vi "MNIST_Optical_int_(SGD)_WB con__v2.2.vi"() -> ()   [LabVIEW 2021]
uses:
  <vilib>/Utility/file.llb/Write Delimited Spreadsheet (I64).vi
  <vilib>/Utility/file.llb/Write Delimited Spreadsheet (DBL).vi
  <vilib>/Utility/file.llb/Read Delimited Spreadsheet (I64).vi
panel:
  in  "WB convert?":bool
  in  "Save? (MiniBatch rows)":bool=TRUE
  in  "Add_in MNIST Rows":string="_MNIST_row_"
  in  "Save? (MiniBatch Num)":bool=TRUE
  in  "Add_in MNIST Num":string="_MNIST_Num_"
  out "Loss":ext
  in  "Save? (EL)":bool=TRUE
  in  "Add_in Erorrs":string="_Errors_"
  in  "Save? (AL)":bool=TRUE
  in  "Add_in Acc&Loss":string="_AL_"
  out "Loss":cluster{i32[], ext[]}(graph)={[1, 2], [45.514396123094795724, nan]}
  in  "Wait2 (ms)":u32=50
  out "Gaussian1 2":dbl[](graph)=[0.09670196140902938, 0.11442214309990176, 0.1351797003320732, 0.15945549418149738, 0.18779935795926087, 0.22083877294599188, 0.2592884397890202, 0.3039608080611435, 0.3557776262498078, 0.41578257333843466, 0.4851550310208827, 0.5652250523124651, 0.657489577737682, 0.7636299442341417, 0.8855307242605183, 1.0252999231821531, 1.1852905516835754, 1.3681235765830648, 1.5767122378728002, 1.8142877019668504, 2.08442600091682, 2.3910761846854314, 2.7385895884155467, 3.131750088996824, 3.57580519515535, 4.076497782861314, 4.640098253206141, 5.273436853240591, 5.983935861846952, 6.779641302867088, 7.669253806815572, 8.662158201039357, 9.768451366679242, 10.99896785985421, 12.365302754810589, 13.879831129103666, 15.555723576025287, 17.406957098330608, 19.448320710770176, 21.69541505796304, 24.164645339736463, 26.873206829207685, 29.83906227058617, 33.0809104548975, 36.61814529350236, 40.470804742262374, 44.65950897426188, 49.20538725679313, 54.12999305937387, 59.45520700425477, 65.20312736937558, 71.39594796601034, 78.05582333916168, 85.2047213776204, 92.86426357174314, 101.05555331939847, 109.79899285287111, 119.11408954021445, 129.01925250173178, 139.53158067379627, 150.66664364569763, 162.4382567879829, 174.85825237998242, 187.93624862685874, 201.6794186294016, 216.0922615296473, 231.1763781989189, 246.93025395874426, 263.3490509260849, 280.424412649283, 298.14428374720154, 316.49274727852463, 335.44988254878865, 354.99164600746684, 375.0897777948495, 395.7117363675348, 416.82066346163936, 438.37538144448484, 460.3304248592841, 482.63610768466145, 505.2386275137416, 528.0802075087822, 551.0992766102449, 574.2306880778159, 597.4059760197224, 620.5536491308751, 643.5995204154158, 666.4670712211182, 689.0778474680089, 711.3518855179752, 733.2081647125599, 754.5650832091166, 775.3409533774449, 795.4545126860733, 814.8254457153614, 833.3749126888666, 851.0260797197676, 867.7046458296478, 883.3393617159861, 897.8625352247819, 911.2105185274822, 923.3241721074656, 934.149300830448, 943.6370576040389, 951.7443104220167, 958.4339689354637, 963.6752670915627, 967.4439988266017, 969.7227042867535, 970.5008045720157, 969.7746835482575, 967.5477158420546, 963.8302407150543, 958.6394821008861, 951.9994156699714, 943.9405843578882, 934.4998643433248, 923.7201839845574, 911.6501987117265, 898.3439253194533, 883.8603395047159, 868.2629408433546, 851.6192896909191, 834.0005207265273, 815.4808380296865, 796.1369966882987, 776.0477759809958, 755.2934491591791, 733.9552547752518, 712.1148743660126, 689.8539211073784, 667.253443812555, 644.3934503552997, 621.3524542682865, 598.2070478996438, 575.0315051146013, 551.8974161102901, 528.873356476583, 506.0245921909981, 483.4128217875633, 461.0959564943735, 439.1279386983413, 417.5585986738939, 396.43354911021174, 375.7941165936193, 355.6773088519376, 336.115816249367, 317.1380457365506, 298.7681852129464, 281.0262960489612, 263.9284313442493, 247.48677736631487, 231.709815519667, 216.60250213925784, 202.16646338132895, 188.4002024981488, 175.2993168281445, 162.85672190694973, 151.06288020502143, 139.9060321206019, 129.37242699969255, 119.44655211405521, 110.11135770074489, 101.3484763490417, 93.13843520969536, 85.46085969410542, 78.29466752455427, 71.61825218825167, 65.40965503532775, 59.646725441864234, 54.30726863171807, 49.36918091364827, 44.810572241806135, 40.60987614694352, 36.745947211971774, 33.19814637826082, 29.94641446804717, 26.971334393482046, 24.254182594381085, 21.776970304983546, 19.522475295517197, 17.474264767749766, 15.616710105755313, 13.934994194693601, 12.41511202241696, 11.043865272147123, 9.80885160030031, 8.69844927277758, 7.701797806667482, 6.8087752332916445, 6.009972563782131, 5.296666000789356, 4.660787400295918, 4.094893446609467, 3.5921339621107853, 3.1462197318544955, 2.751390182199411, 2.4023812127511532, 2.0943934424259196, 1.8230610937190317]
  out "Gaussian1":dbl[](graph)=[0.5699152503773883, 0.6314492251008037, 0.6989600685377171, 0.7729511904764719, 0.853960042130039, 0.9425595629244234, 1.0393596017692057, 1.1450083015934553, 1.2601934350188855, 1.3856436781332593, 1.5221298084293, 1.6704658120969746, 1.831509885009732, 2.0061653109390867, 2.1953811997776564, 2.400153067860802, 2.6215232418633736, 2.8605810672237024, 3.1184629016252225, 3.3963518737600005, 3.695477387421891, 4.017114350943006, 4.362582112109385, 4.733243078982677, 5.130501007526851, 5.555798937604037, 6.0106167597722555, 6.496468396399691, 7.014898581913567, 7.567479228533548, 8.155805365605005, 8.781490642649525, 9.446162388490219, 10.15145622128628, 10.899010207021403, 11.690458566928344, 12.527424937487345, 13.41151518999903, 14.344309820286899, 15.327355922814016, 16.362158767381846, 17.450173000593374, 18.5927934983811, 19.791345900093123, 21.047076858867005, 22.361144047264876, 23.73460596135841, 25.168411570599666, 26.66338986485152, 28.220239353838334, 29.839517577968138, 31.521630692929637, 33.266823193633265, 35.0751678459036, 36.94655589679441, 38.88068763644488, 40.877063385986645, 42.93497498710372, 45.05349786940917, 47.23148377179553, 49.46755419331591, 51.760094647931396, 54.10724979559787, 56.506919519648946, 58.95675601724929, 61.45416196584334, 63.996289824009004, 66.58004231995741, 69.20207417511158, 71.85879510377347, 74.54637412288272, 77.26074519831532, 79.99761424611384, 82.75246749853183, 85.52058123587125, 88.29703287585642, 91.07671340279033, 93.85434110905102, 96.62447661168733, 99.38153909704506, 102.11982373658174, 104.83352020739565, 107.51673224159532, 110.16349811954991, 112.7678120133866, 115.32364607891411, 117.82497318654511, 120.26579017483816, 122.64014150406159, 124.94214318176782, 127.16600682782045, 129.30606374269755, 131.35678884025123, 133.3128243044793, 135.1690028292909, 136.92037030074718, 138.5622077828464, 140.09005267059928, 141.49971887790022, 142.78731593252587, 143.94926685645228, 144.98232471654234, 145.8835877384628, 146.65051288539, 147.28092781258692, 147.77304111920574, 148.12545082960688, 148.33715104799708, 148.40753674217896, 148.3364066245716, 148.12396411130277, 147.7708163529763, 147.27797134357863, 146.6468331267909, 145.87919513161353, 144.9772316815739, 143.94348773377754, 142.78086691557044, 141.49261793751415, 140.08231947164353, 138.5538635934956, 136.911437895094, 135.1595063838758, 133.30278928940297, 131.34624190555502, 129.29503260072028, 127.15452013225598, 124.93023040416011, 122.6278328084785, 120.2531162914655, 117.81196528493653, 115.31033564162118, 112.75423071067677, 110.14967768589845, 107.50270435461167, 104.81931636981285, 102.10547516190402, 99.36707659940957, 96.60993050045434, 93.83974108859331, 91.06208847790437, 88.28241126317056, 85.50599028157492, 82.73793360269933, 79.98316279384422, 77.24640049785856, 74.53215935087066, 71.8447322576235, 69.1881840326221, 66.56634440606591, 63.98280238463786, 61.4409019487149, 58.943739059510534, 56.494159942108, 54.09476060333887, 51.74788753704222, 49.45563956343463, 47.21987074415553, 45.04219431004106, 42.92398753483382, 40.866397484856755, 38.87034757216636, 36.936544836841676, 35.065487882847584, 33.25747539131333, 31.51261513506436, 29.830833418809526, 28.211884870481356, 26.655362510820165, 25.16070803034281, 23.727222205302944, 22.35407538708896, 21.040318002674137, 19.78489100718638, 18.586636233356952, 17.444306586495248, 16.3565760376754, 15.322049371967854, 14.339271652764877, 13.40673736749281, 12.522899224239719, 11.686176573019994, 10.894963429515084, 10.14763608314326, 9.442560275193749, 8.778097936489429, 8.152613477595633, 7.564479627954442, 7.012082823478275, 6.493828145073044, 6.008143813270019, 5.553485246621279, 5.128338693752555, 4.731224450967974, 4.360699679065516, 4.015360834552515, 3.6938457317528375, 3.394835253378139, 3.117054728003027, 2.8592749935482025, 2.620313166346684, 2.3990331356583474, 2.194345803619269, 2.005209090577634, 1.8306277255905967, 1.6696528415498544, 1.521381393981185, 1.3849554220385487, 1.259561169599107, 1.1444280836752243, 1.0388277066049971, 0.9420724776763157, 0.8535144589920913, 0.7725439995066742, 0.6985883502657112, 0.6311102429727983, 0.569606443094855, 0.5136062878118027, 0.46267021822177495, 0.4163883143369015, 0.3743788405519984, 0.33628680844400993, 0.3017825629676108, 0.270560397355318, 0.24233720131135278, 0.21685114640935305, 0.1938604119662967, 0.17314195406955885, 0.15449031988137882, 0.13771650883509554, 0.12264688187001148, 0.10912211942590293, 0.09699622853300671, 0.08613559898751195, 0.07641810829465917, 0.06773227478986307, 0.05997645811098017, 0.053058105990058196, 0.04689304615861079, 0.04140482201462393, 0.03652407058005483, 0.03218794118245605, 0.028339553221509016, 0.02492749132866501, 0.021905336193819215, 0.01923122931509139, 0.016867469924549863, 0.014780142352357088, 0.012938772112715328, 0.011316009025602454]
  in  "SGD?":bool
  in  "Save? (SP)":bool=TRUE
  in  "Add_in Spectrum":string="_spectrum_"
  out "Accuracy(current)":dbl=0.3076923076923077
  out "Errors(current)":i32=36
  out "weight No.":i32=7
  out "epoch":i32=2
  out "Output (Converted)":dbl[](graph)=[39.62523093192144, 0.0, 23.097154266476934, 78.25935170802192, 80.61297751490206, 88.079328272374, 139.1328670628771, 91.58552612543261, 147.85235008560898, 50.15605743167636]
  out "from Start Acq":u32=20002
  out "Waveform Graph 0":i32[](graph)=[148, 148, 147, 146, 147, 147, 149, 149, 148, 148, 146, 147, 146, 149, 148, 148, 148, 149, 148, 147, 148, 147, 148, 146, 150, 149, 148, 147, 148, 147, 148, 148, 147, 149, 147, 145, 149, 148, 148, 146, 148, 148, 146, 148, 150, 150, 147, 148, 150, 147, 146, 148, 148, 147, 146, 151, 151, 153, 149, 149, 148, 150, 149, 151, 152, 151, 149, 149, 150, 150, 150, 150, 150, 154, 150, 152, 153, 152, 152, 152, 155, 155, 153, 154, 156, 155, 156, 159, 159, 161, 163, 161, 161, 163, 161, 165, 168, 168, 167, 169, 172, 178, 175, 176, 179, 178, 184, 186, 186, 188, 190, 194, 200, 200, 200, 200, 206, 205, 207, 212, 220, 222, 219, 221, 227, 231, 234, 233, 237, 244, 247, 246, 253, 257, 262, 259, 266, 270, 273, 279, 279, 281, 280, 284, 292, 291, 301, 297, 298, 301, 307, 303, 300, 306, 303, 309, 307, 305, 303, 307, 303, 307, 300, 301, 295, 288, 291, 289, 286, 280, 279, 280, 271, 270, 264, 268, 264, 260, 262, 251, 250, 251, 248, 241, 236, 240, 233, 230, 230, 232, 225, 224, 225, 220, 223, 219, 216, 221, 213, 212, 205, 210, 206, 202, 203, 201, 203, 198, 197, 202, 194, 195, 193, 196, 187, 191, 188, 187, 184, 183, 184, 181, 181, 178, 178, 179, 178, 173, 176, 175, 177, 174, 171, 174, 170, 172, 171, 170, 168, 166, 169, 169, 168, 163, 167, 165, 162, 162, 164, 163, 163, 162, 161, 163, 159, 161, 163, 162, 159, 157, 156, 157, 156, 158, 158, 155, 155, 153, 155, 156, 154, 155, 155, 151, 151, 153, 151, 152, 151, 150, 150, 151, 150, 151, 151, 151, 151, 150, 148, 151, 148, 150, 149, 149, 149, 149, 148, 149, 148, 148, 150, 150, 150, 149, 149, 150, 150, 149, 148, 152, 150, 150, 149, 148, 150, 149, 150, 147, 150, 151, 150, 150, 149, 149, 147, 149, 147, 149, 149, 149, 148, 151, 150, 148, 149, 150, 151, 149, 149, 150, 152, 150, 150, 150, 148, 148, 148, 149, 149, 147, 147, 148, 150, 150, 148, 149, 149, 149, 148, 149, 147, 149, 152, 149, 148, 150, 149, 149, 150, 150, 150, 148, 151, 150, 150, 148, 150, 149, 150, 147, 149, 152, 150, 148, 149, 148, 150, 149, 149, 149, 149, 150, 149, 149, 151, 148, 150, 150, 152, 149, 151, 151, 149, 146, 150, 148, 148, 149, 150, 148, 149, 150, 148, 149, 148, 150, 148, 150, 150, 149, 150, 150, 147, 152, 148, 150, 150, 149, 151, 149, 150, 148, 149, 149, 149, 149, 148, 147, 150, 149, 149, 151, 151, 151, 148, 150, 148, 150, 151, 149, 149, 147, 151, 150, 147, 149, 149, 150, 150, 149, 149, 151, 149, 149, 149, 150, 148, 152, 149, 150, 150, 151, 149, 149, 149, 148, 149, 149, 149, 149, 148, 149, 148, 149, 150, 150, 148, 149, 150, 149, 149, 148, 151, 150, 149, 151, 148, 148, 149, 147, 150, 151, 148, 151, 150, 150, 149, 148, 149, 150, 150, 149, 149, 151, 148, 148, 151, 151, 148, 148, 149, 150, 151, 149, 151, 152, 151, 151, 150, 151, 151, 151, 149, 148, 148, 150, 152, 152, 148, 152, 151, 151, 150, 150, 151, 151, 151, 151, 153, 152, 151, 153, 153, 152, 153, 155, 153, 154, 155, 151, 153, 156, 154, 154, 154, 156, 155, 156, 157, 158, 155, 157, 158, 160, 159, 159, 160, 161, 162, 163, 165, 166, 164, 170, 169, 169, 171, 172, 176, 174, 174, 178, 181, 183, 185, 187, 186, 193, 196, 194, 199, 199, 202, 203, 210, 211, 219, 219, 221, 226, 233, 237, 242, 246, 252, 257, 260, 269, 274, 277, 281, 287, 292, 303, 309, 313, 327, 328, 340, 346, 359, 367, 371, 377, 389, 402, 406, 418, 437, 436, 447, 453, 463, 480, 488, 500, 519, 530, 523, 550, 570, 597, 601, 605, 622, 639, 646, 660, 684, 691, 711, 736, 760, 767, 795, 792, 827, 838, 864, 877, 898, 912, 934, 946, 980, 991, 1021, 1041, 1053, 1067, 1064, 1089, 1100, 1120, 1125, 1134, 1153, 1155, 1150, 1134, 1151, 1151, 1142, 1126, 1109, 1108, 1100, 1069, 1045, 1015, 987, 971, 934, 904, 875, 844, 816, 793, 760, 731, 704, 680, 651, 619, 587, 575, 549, 516, 510, 488, 473, 456, 436, 414, 403, 393, 381, 357, 348, 339, 329, 324, 311, 299, 292, 286, 276, 271, 267, 257, 253, 246, 241, 231, 233, 227, 224, 216, 214, 209, 209, 202, 201, 200, 197, 195, 191, 186, 187, 184, 184, 179, 180, 178, 173, 176, 176, 169, 174, 169, 167, 170, 167, 171, 167, 167, 166, 164, 164, 161, 162, 161, 161, 158, 161, 157, 160, 157, 160, 157, 155, 157, 156, 155, 156, 155, 155, 155, 153, 154, 154, 153, 154, 155, 154, 154, 154, 152, 152, 153, 150, 152, 154, 153, 153, 150, 152, 152, 150, 150, 153, 150, 149, 149, 151, 151, 151, 151, 150, 151, 150, 150, 151, 152, 150, 148, 150, 152, 151, 150, 149, 149, 150, 149, 151, 148, 150, 150, 149, 149, 150, 148, 151, 151, 148, 149, 150, 150, 149, 149, 149, 149, 151, 147, 149, 149, 149, 146, 151, 151, 150, 148, 147, 151, 149, 149, 147, 151, 147, 148, 150, 147, 148, 148, 149, 150, 147, 148, 148, 150, 148, 150, 148, 149, 148, 150, 148, 147, 147, 146, 150, 149, 149, 150, 147, 150, 149, 148, 150, 149, 149, 148, 148, 149, 148, 147, 149, 149, 147, 149, 148, 147, 146, 149, 148, 149, 147, 147, 147, 149, 148, 147, 149, 149, 150, 147, 147, 149, 151, 150, 148, 148, 148, 146, 147, 149, 148, 146, 149, 148, 147, 149, 147, 148, 149, 149, 147, 147, 148, 149, 149, 146, 149, 147, 150, 147, 148, 149, 149, 148, 149, 148, 149, 148, 148, 150, 148, 149, 148, 147, 148, 147, 147, 149, 148, 149, 148, 147, 148, 147, 148, 148, 147, 149, 148, 147, 148, 150, 148, 147, 147, 150, 147, 147, 147, 148, 148, 149, 149, 147, 146, 147, 149, 150, 147, 146, 149, 149, 148, 146, 146, 149, 147, 148]
  in  "Ind1":i32=50
  in  "Leng1":i32=250
  in  "Ind2":i32=575
  in  "Leng2":i32=200
  in  "Compen_Factor":dbl=3.0
  out "In * W (i) +B (i)":dbl[][](graph)
  in  "Wait1 (ms)":u32=50
  out "Weights(i)":dbl[][](graph)=[[25.0, 75.0, 53.0, -76.0, -17.0, -21.0, -83.0, 41.0, -26.0, -83.0, -71.0, -83.0, 76.0, -65.0, 57.0, 83.0, -8.0, 41.0, -28.0, 67.0, 47.0, 31.0, -41.0, 72.0, -83.0, 81.0, -16.0, -24.0], [5.0, -71.0, 45.0, 74.0, 50.0, -18.0, -76.0, 28.0, -37.0, -41.0, -28.0, 2.0, -20.0, -69.0, 53.0, 83.0, 10.0, -70.0, 83.0, -53.0, -49.0, 56.0, 53.0, -3.0, -83.0, -57.0, -76.0, 56.0], [44.0, -79.0, 83.0, 51.0, 30.0, 46.0, 12.0, 41.0, 3.0, -20.0, -50.0, 83.0, -50.0, 83.0, -36.0, -65.0, -76.0, -52.0, 25.0, -17.0, 21.0, 23.0, -29.0, 15.0, 80.0, 70.0, 19.0, -83.0], [-65.0, -83.0, -83.0, 38.0, -7.0, 41.0, 44.0, 50.0, 80.0, 23.0, 34.0, -5.0, 83.0, -12.0, 0.0, -14.0, -2.0, -25.0, -83.0, 40.0, -62.0, -83.0, 56.0, -83.0, 83.0, -4.0, 48.0, 25.0], [-83.0, -83.0, 65.0, -41.0, -71.0, -81.0, -8.0, -45.0, 41.0, -76.0, -32.0, -56.0, 41.0, -78.0, -83.0, -83.0, 23.0, -74.0, 17.0, -15.0, -72.0, 41.0, -83.0, 41.0, 44.0, 83.0, -57.0, -83.0], [-83.0, -28.0, 8.0, 81.0, 71.0, 78.0, -3.0, -79.0, -10.0, -83.0, -21.0, 10.0, 21.0, -86.0, -8.0, -56.0, -3.0, -90.0, -25.0, -52.0, -2.0, 19.0, -43.0, -59.0, 49.0, 83.0, 37.0, -28.0], [5.0, 52.0, -83.0, -12.0, -34.0, 32.0, -42.0, -53.0, -50.0, -87.0, -52.0, -18.0, -89.0, 76.0, -26.0, 10.0, 23.0, 5.0, -83.0, -33.0, 36.0, -60.0, 1.0, -32.0, -83.0, 83.0, -58.0, -12.0], [17.0, -41.0, -59.0, 38.0, -8.0, 39.0, 71.0, -15.0, 76.0, 18.0, 87.0, -78.0, -6.0, 75.0, 49.0, -43.0, 25.0, 39.0, 58.0, -42.0, -76.0, -83.0, -9.0, 83.0, 55.0, -21.0, -83.0, 23.0], [-83.0, -83.0, 29.0, 81.0, 36.0, 94.0, 20.0, 106.0, 38.0, 1.0, 99.0, 90.0, -25.0, 10.0, 107.0, 70.0, 91.0, 101.0, -3.0, 103.0, -14.0, -34.0, -83.0, -58.0, 1.0, -83.0, -5.0, 11.0], [65.0, 85.0, 25.0, 83.0, 32.0, 24.0, -65.0, 43.0, -29.0, 93.0, 108.0, -15.0, 26.0, 103.0, 50.0, 115.0, 125.0, 75.0, 113.0, -17.0, 6.0, -37.0, -28.0, -83.0, 36.0, -7.0, 62.0, -8.0], [56.0, -36.0, 80.0, -32.0, 64.0, 35.0, 90.0, 25.0, 52.0, 87.0, 106.0, 72.0, 101.0, -59.0, 47.0, 115.0, 110.0, 71.0, 106.0, 113.0, 81.0, 98.0, 86.0, -63.0, 83.0, 83.0, 36.0, 33.0], [24.0, 6.0, 9.0, -41.0, 50.0, -18.0, 56.0, 65.0, 87.0, -42.0, 103.0, 19.0, 28.0, -79.0, -17.0, 83.0, 48.0, 112.0, 110.0, 99.0, 66.0, 95.0, 5.0, -18.0, -77.0, -41.0, -71.0, 83.0], [9.0, -36.0, 26.0, 83.0, 41.0, 5.0, 39.0, -17.0, 101.0, -13.0, 45.0, 50.0, -69.0, -74.0, -10.0, -40.0, -12.0, -32.0, 65.0, -11.0, 41.0, -37.0, 23.0, 40.0, 0.0, 23.0, 62.0, -80.0], [40.0, -39.0, 83.0, 74.0, -61.0, 6.0, -14.0, -1.0, -9.0, 53.0, -14.0, -158.0, -125.0, -96.0, 32.0, 9.0, -63.0, 60.0, -32.0, -23.0, 74.0, 26.0, 74.0, 83.0, 83.0, -42.0, -56.0, 83.0], [-83.0, -3.0, 67.0, 59.0, 26.0, 82.0, 2.0, 84.0, 15.0, -87.0, -90.0, -135.0, -113.0, -92.0, -58.0, -24.0, 77.0, 109.0, -13.0, 94.0, -12.0, 38.0, 32.0, -3.0, 40.0, 35.0, -35.0, 17.0], [81.0, 37.0, 38.0, 30.0, -37.0, 34.0, 3.0, -54.0, 59.0, -98.0, -31.0, -60.0, -127.0, -45.0, -70.0, 20.0, 76.0, 61.0, 40.0, -8.0, -32.0, 35.0, -76.0, 46.0, 86.0, -50.0, -17.0, 83.0], [28.0, -53.0, 19.0, 18.0, -78.0, 3.0, 65.0, -59.0, 85.0, 86.0, -32.0, -40.0, 0.0, 41.0, -46.0, 68.0, 21.0, 97.0, 99.0, -65.0, -65.0, 4.0, -6.0, -83.0, -83.0, 75.0, 0.0, 61.0], [65.0, -83.0, 78.0, -44.0, -41.0, -83.0, -33.0, -63.0, 7.0, 25.0, -76.0, -22.0, -16.0, -2.0, 124.0, 15.0, 50.0, -68.0, -14.0, 68.0, -87.0, -55.0, -81.0, -26.0, 2.0, -65.0, 19.0, -14.0], [15.0, -41.0, -15.0, -68.0, -55.0, 39.0, 74.0, -52.0, 79.0, -37.0, -71.0, -8.0, -15.0, 95.0, 88.0, 70.0, 12.0, 41.0, -52.0, 43.0, -86.0, -87.0, -85.0, -64.0, 41.0, -80.0, 23.0, -79.0], [69.0, 25.0, -65.0, 83.0, 33.0, -32.0, -83.0, -36.0, -80.0, -36.0, 18.0, 37.0, -15.0, 36.0, 38.0, 110.0, -45.0, -80.0, -57.0, 31.0, -19.0, -22.0, -56.0, 83.0, -83.0, 3.0, -28.0, -83.0], [-35.0, 83.0, 74.0, 38.0, -26.0, 83.0, 48.0, 44.0, -83.0, 65.0, 46.0, -24.0, 12.0, 23.0, -58.0, 25.0, -29.0, -49.0, 41.0, 42.0, 38.0, -57.0, 11.0, 17.0, -76.0, -15.0, -48.0, 72.0], [83.0, -83.0, -67.0, -57.0, 83.0, 83.0, -79.0, -14.0, 72.0, -78.0, -71.0, -74.0, -26.0, 98.0, 103.0, -28.0, -20.0, 17.0, -85.0, -17.0, -85.0, -54.0, -85.0, -17.0, -57.0, 6.0, -80.0, -76.0], [-83.0, 67.0, 64.0, -56.0, 76.0, 71.0, 46.0, -69.0, -37.0, 68.0, 14.0, 19.0, -32.0, -35.0, -37.0, 55.0, 11.0, -46.0, 19.0, -28.0, 30.0, -8.0, 60.0, 9.0, 41.0, 36.0, -31.0, -83.0], [42.0, 57.0, -50.0, 83.0, -71.0, -72.0, 83.0, 0.0, 87.0, -57.0, 48.0, 91.0, -76.0, -40.0, 5.0, 62.0, -50.0, -79.0, -25.0, -41.0, 32.0, 1.0, 83.0, 6.0, -83.0, -52.0, -72.0, 7.0], [41.0, 53.0, -76.0, -74.0, 62.0, -44.0, -1.0, 52.0, 20.0, 85.0, 92.0, 41.0, 54.0, 9.0, 114.0, 82.0, -81.0, 46.0, -49.0, -79.0, -74.0, 43.0, -28.0, -83.0, 26.0, -30.0, 83.0, 83.0], [-57.0, -83.0, 23.0, 52.0, -25.0, 49.0, -28.0, 22.0, -34.0, 42.0, 32.0, -11.0, 82.0, 99.0, 99.0, -25.0, 58.0, 52.0, -65.0, 83.0, 53.0, 32.0, 56.0, -43.0, 61.0, 25.0, -83.0, -32.0], [-77.0, 83.0, 80.0, 37.0, 33.0, -83.0, 3.0, 24.0, 90.0, -17.0, -45.0, -78.0, 97.0, 80.0, 36.0, 73.0, 53.0, 68.0, 83.0, -41.0, 83.0, -66.0, -83.0, 14.0, -79.0, 59.0, -83.0, 83.0], [-35.0, -83.0, 48.0, 78.0, 47.0, 13.0, -79.0, 30.0, -64.0, -5.0, 36.0, -39.0, 50.0, -26.0, -83.0, -8.0, -51.0, -25.0, 77.0, -56.0, 21.0, -83.0, -11.0, -41.0, -41.0, 57.0, 81.0, -44.0], [-71.0, 0.0, 0.0, 0.0, 0.0, 0.0, 0.0, 0.0, 0.0, 0.0, 0.0, 0.0, 0.0, 0.0, 0.0, 0.0, 0.0, 0.0, 0.0, 0.0, 0.0, 0.0, 0.0, 0.0, 0.0, 0.0, 0.0, 0.0]]
  in  "WB Import?":bool=TRUE
  out "Output (Measured)":dbl[](graph)=[792.5046186384288, -931.6896199556032, 461.9430853295387, 1565.1870341604385, 1612.2595502980412, 1761.58656544748, 2782.6573412575417, 1831.710522508652, 2957.0470017121793, 1003.1211486335272]
  in  "Epochs":i64=200
  out "Accu":cluster{i32[], dbl[]}(graph)={[1, 2], [0.29, 0.14]}
  in  "Training rate":dbl=2.0 format="%#_13g"
  in  "Con.F":i32=20
  out "min value":i32=-255
  out "max value":i32=176
  in  "Add_in WB":string="_epoch__"
  out "W&B(int)":i32[][](array[numeric])
  out "Output (simulated)":dbl[](graph)=[-161692.0, -526023.0, -407243.0, 774561.0, -189118.0, -52721.0, -448721.0, 622480.0, 408514.0, -270311.0]
  out "Output (SoftMax)":ext[](graph)=[9.942335489197921718e-48, 6.1442556256622408318e-65, 6.5983587063865749592e-55, 5.9713685974966820238e-31, 6.2840637228245183395e-30, 1.0985896780412405855e-26, 0.000163344942582687903655, 3.6606473610987689061e-25, 0.99983665505741731205, 3.7236448483001870884e-43]
  out "No. Tested":i32=53
  out "Accuracy (prev)":dbl=0.14
  out "Errors":i32=86
  out "Error list":i32[][](array[numeric])=[[0, 2, 3, 5, 6, 7, 8, 9, 10, 11, 12, 13, 14, 15, 16, 17, 18, 20, 22, 23, 24, 25, 26, 27, 28, 29, 30, 31, 32, 33, 34, 35, 36, 38, 39, 40, 41, 42, 43, 44, 45, 46, 47, 48, 49, 50, 52, 53, 54, 55, 57, 58, 59, 60, 61, 62, 64, 65, 66, 67, 70, 71, 72, 73, 74, 76, 77, 78, 79, 80, 82, 83, 84, 85, 86, 87, 89, 90, 91, 92, 93, 94, 96, 97, 98, 99], [5, 4, 1, 2, 1, 3, 1, 4, 3, 5, 3, 6, 1, 7, 2, 8, 6, 4, 9, 1, 1, 2, 4, 3, 2, 7, 3, 8, 6, 9, 0, 5, 6, 7, 6, 1, 8, 7, 9, 3, 9, 8, 5, 9, 3, 3, 7, 4, 9, 8, 9, 4, 1, 4, 4, 6, 4, 5, 6, 1, 1, 7, 1, 6, 3, 2, 1, 1, 7, 9, 2, 6, 7, 8, 3, 9, 4, 6, 7, 4, 6, 8, 7, 8, 3, 1], [0, 0, 9, 0, 9, 0, 9, 9, 0, 1, 0, 0, 9, 0, 0, 1, 1, 9, 1, 9, 0, 8, 9, 0, 0, 9, 0, 9, 0, 0, 1, 0, 1, 0, 0, 9, 1, 9, 0, 0, 0, 9, 1, 0, 0, 0, 0, 9, 0, 9, 0, 9, 9, 9, 9, 1, 0, 1, 1, 9, 0, 0, 9, 1, 0, 1, 9, 9, 0, 0, 0, 0, 0, 1, 0, 0, 0, 0, 0, 0, 9, 9, 0, 1, 0, 9]]
  out "Match?":bool
  in  "Train No.":i32=10
  out "OUTPUT":i16=8
  out "MNIST_Input":i32[][](graph)=[[0, 0, 0, 0, 0, 0, 0, 0, 0, 0, 0, 0, 0, 0, 0, 0, 0, 0, 0, 0, 0, 0, 0, 0, 0, 0, 0, 0], [0, 0, 0, 0, 0, 0, 0, 0, 0, 0, 0, 0, 0, 0, 0, 0, 0, 0, 0, 0, 0, 0, 0, 0, 0, 0, 0, 0], [0, 0, 0, 0, 0, 0, 0, 0, 0, 0, 0, 0, 0, 0, 0, 0, 0, 0, 0, 0, 0, 0, 0, 0, 0, 0, 0, 0], [0, 0, 0, 0, 0, 0, 0, 0, 0, 0, 0, 0, 0, 0, 0, 0, 0, 0, 0, 0, 0, 0, 0, 0, 0, 0, 0, 0], [0, 0, 0, 0, 0, 0, 0, 0, 0, 0, 0, 0, 0, 0, 0, 0, 0, 0, 0, 0, 0, 0, 0, 0, 0, 0, 0, 0], [0, 0, 0, 0, 0, 0, 0, 0, 0, 0, 0, 0, 0, 0, 0, 0, 0, 0, 0, 0, 0, 0, 0, 0, 0, 0, 0, 0], [0, 0, 0, 0, 0, 0, 0, 0, 0, 0, 0, 0, 0, 0, 0, 0, 0, 0, 0, 0, 0, 0, 0, 0, 0, 0, 0, 0], [0, 0, 0, 0, 0, 0, 0, 1, 109, 109, 109, 109, 110, 109, 129, 253, 110, 109, 31, 0, 0, 0, 0, 0, 0, 0, 0, 0], [0, 0, 0, 0, 0, 21, 94, 217, 252, 252, 252, 252, 253, 252, 252, 252, 253, 252, 227, 134, 42, 0, 0, 0, 0, 0, 0, 0], [0, 0, 0, 0, 0, 176, 252, 252, 252, 252, 252, 252, 253, 252, 252, 252, 253, 252, 252, 252, 222, 139, 11, 0, 0, 0, 0, 0], [0, 0, 0, 0, 0, 217, 252, 252, 252, 128, 108, 108, 108, 108, 108, 108, 108, 232, 252, 252, 253, 252, 71, 0, 0, 0, 0, 0], [0, 0, 0, 0, 0, 42, 159, 252, 252, 210, 31, 0, 0, 0, 0, 0, 0, 0, 37, 252, 253, 252, 71, 0, 0, 0, 0, 0], [0, 0, 0, 0, 0, 0, 5, 119, 210, 252, 124, 31, 0, 0, 0, 0, 0, 0, 37, 252, 253, 231, 51, 0, 0, 0, 0, 0], [0, 0, 0, 0, 0, 0, 0, 0, 31, 195, 195, 31, 0, 0, 0, 0, 0, 0, 140, 252, 253, 158, 0, 0, 0, 0, 0, 0], [0, 0, 0, 0, 0, 0, 0, 0, 0, 0, 0, 0, 0, 0, 0, 0, 0, 42, 221, 252, 191, 15, 0, 0, 0, 0, 0, 0], [0, 0, 0, 0, 0, 0, 0, 0, 0, 0, 0, 0, 0, 0, 0, 0, 0, 218, 253, 253, 84, 0, 0, 0, 0, 0, 0, 0], [0, 0, 0, 0, 0, 0, 0, 0, 0, 0, 0, 0, 0, 0, 0, 0, 94, 247, 252, 210, 0, 0, 0, 0, 0, 0, 0, 0], [0, 0, 0, 0, 0, 0, 0, 0, 0, 0, 0, 0, 0, 0, 0, 21, 212, 252, 226, 31, 0, 0, 0, 0, 0, 0, 0, 0], [0, 0, 0, 0, 0, 0, 0, 0, 0, 0, 0, 0, 0, 0, 0, 144, 253, 252, 132, 0, 0, 0, 0, 0, 0, 0, 0, 0], [0, 0, 0, 0, 0, 0, 0, 0, 0, 0, 0, 0, 0, 0, 99, 253, 255, 222, 41, 0, 0, 0, 0, 0, 0, 0, 0, 0], [0, 0, 0, 0, 0, 0, 0, 0, 0, 0, 0, 0, 0, 21, 201, 252, 253, 55, 0, 0, 0, 0, 0, 0, 0, 0, 0, 0], [0, 0, 0, 0, 0, 0, 0, 0, 0, 0, 0, 0, 0, 94, 252, 252, 175, 10, 0, 0, 0, 0, 0, 0, 0, 0, 0, 0], [0, 0, 0, 0, 0, 0, 0, 0, 0, 0, 0, 0, 0, 217, 252, 252, 62, 0, 0, 0, 0, 0, 0, 0, 0, 0, 0, 0], [0, 0, 0, 0, 0, 0, 0, 0, 0, 0, 0, 0, 171, 253, 253, 170, 110, 78, 0, 0, 0, 0, 0, 0, 0, 0, 0, 0], [0, 0, 0, 0, 0, 0, 0, 0, 0, 0, 0, 0, 253, 252, 252, 252, 253, 55, 0, 0, 0, 0, 0, 0, 0, 0, 0, 0], [0, 0, 0, 0, 0, 0, 0, 0, 0, 0, 0, 0, 253, 252, 252, 252, 154, 10, 0, 0, 0, 0, 0, 0, 0, 0, 0, 0], [0, 0, 0, 0, 0, 0, 0, 0, 0, 0, 0, 0, 253, 252, 252, 168, 0, 0, 0, 0, 0, 0, 0, 0, 0, 0, 0, 0], [0, 0, 0, 0, 0, 0, 0, 0, 0, 0, 0, 0, 0, 0, 0, 0, 0, 0, 0, 0, 0, 0, 0, 0, 0, 0, 0, 0], [255, 0, 0, 0, 0, 0, 0, 0, 0, 0, 0, 0, 0, 0, 0, 0, 0, 0, 0, 0, 0, 0, 0, 0, 0, 0, 0, 0]]
  in  "MNIST_train/test_cvs_file path":path=path "C:/Users/user/NEPL Dropbox/연구실 공용/뉴로모픽 과제/MNIST_Optical_Mea_Program/MNIST data/mnist_train.csv"
  in  "WB_cvs_file":path=path "C:/Users/user/NEPL Dropbox/연구실 공용/뉴로모픽 과제/MNIST_Optical_Mea_Program/weights&Biases/0517/train no.400/WB_100_500Tr.csv"
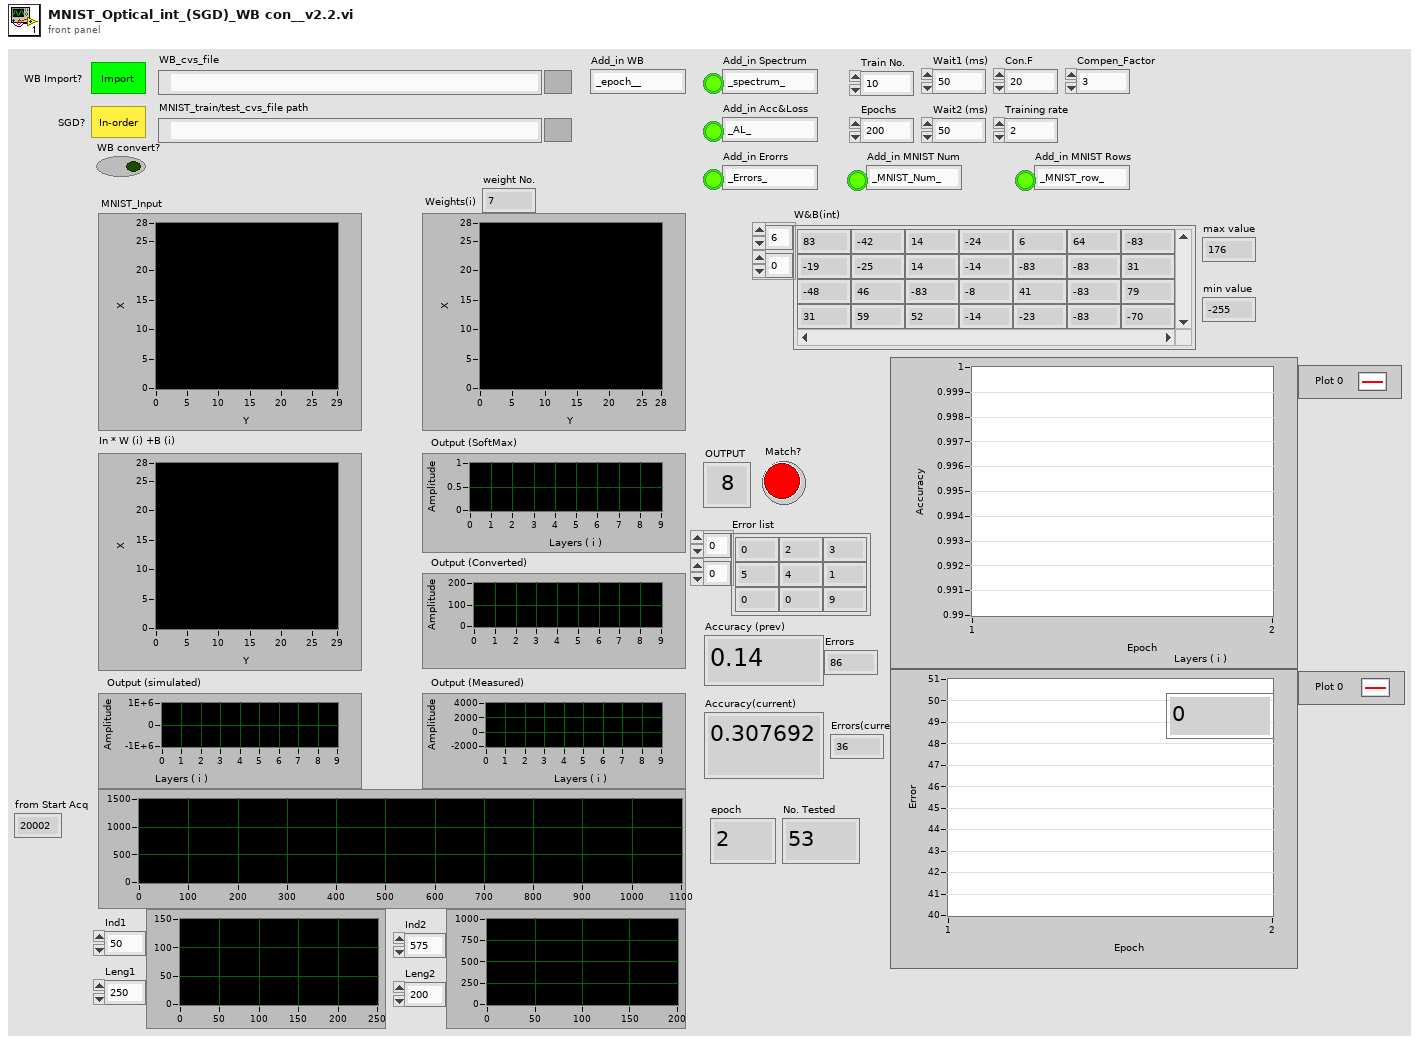
[diagram p1: front panel]
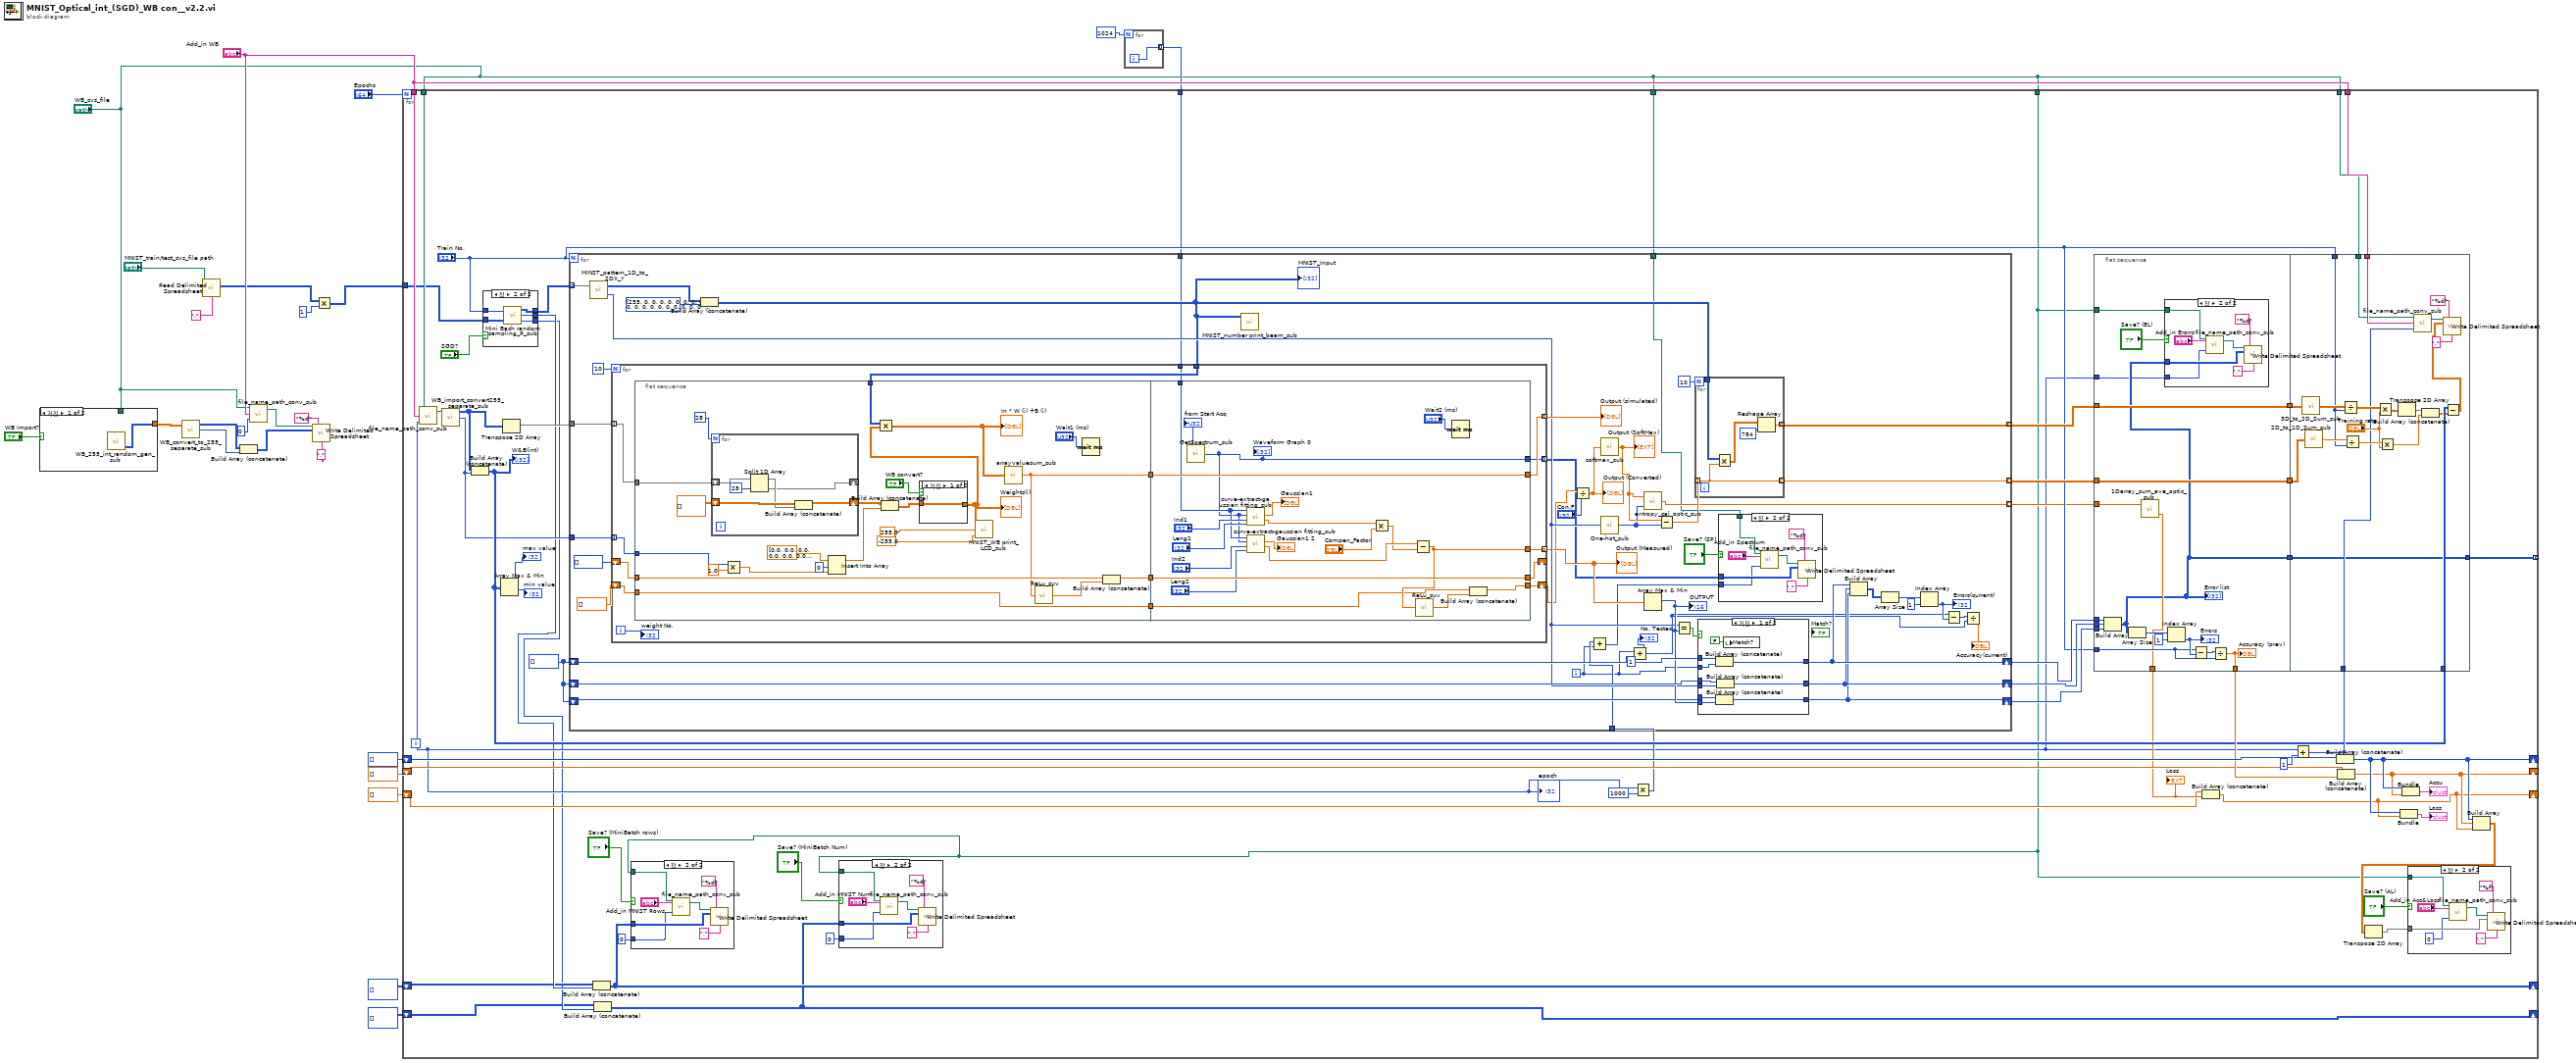
[diagram p0: block diagram]
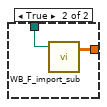
[diagram p2: hidden frame]
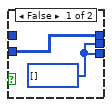
[diagram p6: hidden frame]
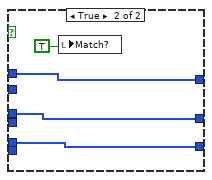
[diagram p9: hidden frame]
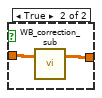
[diagram p10: hidden frame]
diagram:
  n1 = case shown="거짓" "WB Import?" {
    tunnel: [w25 w27] -> w20
    tunnel: "WB_cvs_file" -> [_ w26]
    frame False {
      n2 = call "WB_255_int_random_gen_sub.vi"() -> ("배열"=w25:i64[][])  [unwired: 1 in, 1 out]
    }
    frame True {
      n3 = call "WB_F_import_sub.vi"("Import_weights_cvs"=w26) -> ("WB"=w27:dbl[][])  [unwired: 3 in]
    }
  }
  n4 = call "WB_convert_to_255_separate_sub.vi"("Weights & Biases"=w20) -> ("Biases"=w21:i64[], "Weights"=w22:i64[][])  [unwired: 1 in, 2 out]
  n5 = call-poly <vilib>:"Read Delimited Spreadsheet.vi"("file path (dialog if empty)"="MNIST_train/test_cvs_file path", "delimiter (\\t)"="," ("delimiter (\\t)")) -> ("all rows"=w8:i64[][])  [unwired: 8 in, 5 out]
  n6 = Build Array (concatenate)(w22, w21) -> (w18:i64[][])
  n7 = call "file_name_path_conv_sub.vi"("Add_No"=0, "Add_Str"="Add_in WB", "path_In"="WB_cvs_file") -> ("path_Out"=w17:path)  [unwired: 1 in]
  n8 = call-poly <vilib>:"Write Delimited Spreadsheet.vi"("file path (dialog if empty)"=w17, "format (%d)"="%d", "2D data"=w18, "delimiter (\\t)"="," ("delimiter (\\t)")) -> ()  [unwired: 10 in, 2 out]
  n9 = Multiply(x=w8, y=1) -> (x*y=w7:i64[][])
  n10 = for {
    N: 1024 -> [_]
    tunnel: [w28] -> w5 mode=indexing
    i -> [w28]
  }
  n11 = for {
    N: "Epochs" -> [_]
    tunnel: w7 -> [w59]
    shift-right: [w48] -> _
    shift-left: i32[] [] -> [w71]
    shift-right: [w47] -> _
    shift-left: dbl[] [] -> [w69]
    tunnel: "Add_in WB" -> [w67]
    tunnel: "WB_cvs_file" -> [w66]
    tunnel: "Add_in WB" -> [w65]
    tunnel: "WB_cvs_file" -> [w64]
    tunnel: w5 -> [w56]
    shift-right: [w46] -> _
    shift-left: ext[] [] -> [w51]
    tunnel: "WB_cvs_file" -> [w45]
    tunnel: "WB_cvs_file" -> [w29]
    tunnel: [w44] -> _ mode=indexing
    shift-right: [w33] -> _
    shift-left: i32[][] [] -> [w34]
    shift-right: [w30] -> _
    shift-left: i32[][] [] -> [w31]
    i -> [w42]
    w83 = i32[] []
    n12 = call "file_name_path_conv_sub.vi"("Add_No"=w42, "Add_Str"=w67, "path_In"=w66) -> ("path_Out"=w77:path)  [unwired: 1 in]
    n13 = call "WB_import_convert255_separate_sub.vi"("weights&Biases_cvs_file path"=w77) -> ("Weights"=w63:i64[][], "Biases"=w61:i64[])  [unwired: 2 in, 5 out]
    n14 = Build Array (concatenate)(w63, w61) -> (w62:i64[][])
    "W&B(int)" <- w62
    n15 = case shown="참" "SGD?" {
      tunnel: "Train No." -> [_ w113]
      tunnel: w59 -> [w108 w112]
      tunnel: [w108 w111] -> w57
      tunnel: [w107 w110] -> w32
      tunnel: [w107 w109] -> w35
      frame False {
        w107 = i32[] [] ("MNIST Num")
      }
      frame True {
        n16 = call "Mini Bach random sampling_R_sub.vi"("Mini Bach No."=w113, "MNIST Input"=w112) -> ("MNIST Random Output"=w111:i32[][], "MNIST No.Row"=w109:i32[], "MNIST Num"=w110:i32[])
      }
    }
    n17 = Array Max & Min(array=w62) -> (max value=→"max value":i64, min value=→"min value":i64)  [unwired: 2 out]
    n18 = Transpose 2D Array(2D array=w63) -> (transposed array=w76:i64[][])
    n19 = Build Array (concatenate)(w34, w35) -> (w33:i32[][])
    n20 = Build Array (concatenate)(w31, w32) -> (w30:i32[][])
    n21 = case shown="참" "Save? (MiniBatch rows)" {
      tunnel: w33 -> [_ w89]
      tunnel: w29 -> [_ w87]
      tunnel: 0 -> [_ w86]
      frame False {
      }
      frame True {
        n22 = call "file_name_path_conv_sub.vi"("Add_No"=w86, "Add_Str"="Add_in MNIST Rows", "path_In"=w87) -> ("path_Out"=w90:path)  [unwired: 1 in]
        n23 = call-poly <vilib>:"Write Delimited Spreadsheet.vi"("file path (dialog if empty)"=w90, "format (%d)"="%d", "2D data"=w89, "delimiter (\\t)"="," ("delimiter (\\t)")) -> ()  [unwired: 10 in, 2 out]
      }
    }
    n24 = case shown="참" "Save? (MiniBatch Num)" {
      tunnel: w30 -> [_ w96]
      tunnel: w29 -> [_ w94]
      tunnel: 0 -> [_ w93]
      frame False {
      }
      frame True {
        n25 = call "file_name_path_conv_sub.vi"("Add_No"=w93, "Add_Str"="Add_in MNIST Num", "path_In"=w94) -> ("path_Out"=w97:path)  [unwired: 1 in]
        n26 = call-poly <vilib>:"Write Delimited Spreadsheet.vi"("file path (dialog if empty)"=w97, "format (%d)"="%d", "2D data"=w96, "delimiter (\\t)"="," ("delimiter (\\t)")) -> ()  [unwired: 10 in, 2 out]
      }
    }
    n27 = Multiply(x=w42, y=1000) -> (x*y=w54:i32)
    n28 = for {
      N: "Train No." -> [_]
      tunnel: w76 -> [w203]
      tunnel: w61 -> [w201]
      tunnel: w57 -> [w185] mode=indexing
      shift-right: [w173] -> w82
      shift-left: w83 -> [w198]
      shift-right: [w172] -> w81
      shift-left: w83 -> [w197]
      shift-right: [w171] -> w80
      shift-left: w83 -> [w195]
      tunnel: [w187] -> w75 mode=indexing
      tunnel: [w186] -> w74 mode=indexing
      tunnel: w56 -> [w166]
      tunnel: w54 -> [w165]
      tunnel: [w160] -> w53 mode=indexing
      tunnel: w45 -> [w159]
      i -> [w164]
      n29 = call "MINST_pattern_1D_to_2DX_Y.vi"("pattern 1D"=w185) -> ("Pattern_Y"=w190:i16, "2D(28_28)"=w191:i32[][])  [unwired: 1 in]
      n30 = Build Array (concatenate)(w191, i32[] [255, 0, 0, 0, 0, 0, 0, 0, 0, 0, 0, 0, 0, 0, 0, 0, 0, 0, 0, 0, 0, 0, 0, 0, 0, 0, 0, 0] ("두 번째 부분배열")) -> (w167:i32[][])
      "MNIST_Input" <- w167
      n31 = for {
        N: 10 -> [_]
        tunnel: w203 -> [w241] mode=indexing
        tunnel: w167 -> [w242]
        shift-right: [w237] -> _
        shift-left: i32[] [] -> [w239]
        tunnel: w201 -> [w240] mode=indexing
        tunnel: [w238] -> w192 mode=indexing
        tunnel: [w236] -> w183 mode=indexing
        shift-right: [w235] -> w180
        shift-left: dbl[] [] -> [w233]
        tunnel: [w231] -> w169 mode=indexing
        tunnel: w166 -> [w230]
        i -> [w232]
        n32 = flat-sequence {
          tunnel: w241 -> [w265]
          tunnel: w242 -> [w264]
          tunnel: w239 -> [w262]
          tunnel: w240 -> [w255]
          tunnel: [w263] -> w244
          tunnel: [w252] -> w243
          tunnel: [w251] -> w234
          tunnel: w233 -> [w251]
          tunnel: [w295] -> w238
          tunnel: [w296] -> w237
          tunnel: w244 -> [w296]
          tunnel: w243 -> [w295]
          tunnel: [w291] -> w236
          tunnel: [w290] -> w235
          tunnel: w234 -> [w289]
          tunnel: [w277] -> w231
          tunnel: w230 -> [w286]
          frame #0 {
            n33 = for {
              N: 28 -> [_]
              shift-right: [w275] -> w256
              shift-left: dbl[][] [] -> [w274]
              shift-right: [w272] -> _
              shift-left: w265 -> [w271]
              n34 = Split 1D Array(array=w271, index=28) -> (first subarray=w273:i64[], second subarray=w272:i64[])
              n35 = Build Array (concatenate)(w274, w273) -> (w275:dbl[][])
            }
            n36 = Multiply(x=w255, y=1.0) -> (x*y=w253:dbl)
            n37 = Insert Into Array(array=dbl[] [0.0, 0.0, 0.0, 0.0, 0.0, 0.0, 0.0, 0.0, 0.0, 0.0, 0.0, 0.0, 0.0, 0.0, 0.0, 0.0, 0.0, 0.0, 0.0, 0.0, 0.0, 0.0, 0.0, 0.0, 0.0, 0.0, 0.0] ("두 번째 부분배열"), index=0 ("인덱스"), new element=w253) -> (w257:dbl[])
            n38 = Build Array (concatenate)(w256, w257) -> (w247:dbl[][])
            n39 = case shown="거짓" "WB convert?" {
              tunnel: w247 -> [w268 w270]
              tunnel: [w268 w269] -> w246
              frame False {
              }
              frame True {
                n40 = call "WB_correction_sub.vi"("Input 2D"=w270) -> ("Output 2D 2"=w269:dbl[][])  [unwired: 2 in]
              }
            }
            "Weights(i)" <- w246
            n41 = Multiply(x=w264, y=w246) -> (x*y=w261:dbl[][])
            "In * W (i) +B (i)" <- w261
            n42 = call "MNIST_WB print_LCD_sub.vi"("최소값"=-255.0, "최대값"=255.0, "배열"=w246) -> ()  [unwired: 1 out]
            n43 = call "arrayvaluesum_sub.vi"("all rows 2"=w261) -> ("Numeric"=w252:dbl)
            n44 = call "ReLu_suv.vi"("Input"=w252) -> ("Output"=w260:dbl)
            n45 = Wait (ms)(milliseconds to wait="Wait1 (ms)") -> ()  [unwired: 1 out]
            n46 = Build Array (concatenate)(w262, w260) -> (w263:dbl[])
          }
          frame #1 {
            n47 = call "GetSpectrum_sub.vi"() -> ("array"=w277:i32[], "from Start Acq"=→"from Start Acq":u32)  [unwired: 2 out]
            "Waveform Graph 0" <- w277
            n48 = call "curve-extract-gaussian fitting_sub.vi"("X array"=w286, "Y array"=w277, "index"="Ind1", "length"="Leng1") -> ("Best Gaussian Fit"=→"Gaussian1":dbl[], "amplitude"=w283:dbl)  [unwired: 1 in, 4 out]
            n49 = call "curve-extract-gaussian fitting_sub.vi"("X array"=w286, "Y array"=w277, "index"="Ind2", "length"="Leng2") -> ("Best Gaussian Fit"=→"Gaussian1 2":dbl[], "amplitude"=w279:dbl)  [unwired: 1 in, 4 out]
            n50 = Multiply(x=w283, y="Compen_Factor") -> (x*y=w278:dbl)
            n51 = Subtract(x=w279, y=w278) -> (x-y=w291:dbl)
            n52 = call "ReLu_suv.vi"("Input"=w291) -> ("Output"=w292:dbl)
            n53 = Wait (ms)(milliseconds to wait="Wait2 (ms)") -> ()  [unwired: 1 out]
            n54 = Build Array (concatenate)(w289, w292) -> (w290:dbl[])
          }
        }
        "weight No." <- w232
      }
      "Output (simulated)" <- w192
      "Output (Measured)" <- w183
      n55 = call "MNIST_number print_beam_sub.vi"("배열"=w167) -> ()  [unwired: 2 in, 1 out]
      n56 = Divide(x=w180, y="Con.F") -> (x/y=w182:dbl[])
      "Output (Converted)" <- w182
      n57 = Add(x=w165, y=w164) -> (x+y=w163:i32)
      n58 = call "softmax_sub.vi"("Input"=w182) -> ("Output"=w162:ext[])
      "Output (SoftMax)" <- w162
      n59 = call "One-hot_sub.vi"("Input(Y)"=w190) -> ("Output(One-hot)"=w161:i32[])
      n60 = Add(x=w164, y=1) -> (x+y=w170:i32)
      "No. Tested" <- w170
      n61 = call "entropy_cal_optic_sub.vi"("T_1D"=w161, "Y_1D"=w162) -> ("Entropy"=w160:ext)
      n62 = Array Max & Min(array=w183) -> (max index (indices)=w196:i32)  [unwired: 3 out]
      "OUTPUT" <- w196
      n63 = Subtract(x=w162, y=w161) -> (x-y=w189:ext[])
      n64 = Equal?(x=w190, y=w196) -> (x = y?=w199:bool)
      n65 = for {
        N: 10 -> [_]
        tunnel: w189 -> [w212] mode=indexing
        tunnel: w167 -> [w215]
        tunnel: [w212] -> w186 mode=indexing
        tunnel: [w211] -> w187 mode=indexing
        n66 = Multiply(x=w215, y=w212) -> (x*y=w214:ext[][])
        n67 = Reshape Array(w214, 784 ("차원 크기")) -> (w211:ext[])
      }
      n68 = case shown="거짓" w199 {
        tunnel: w164 -> [w225 _]
        tunnel: [w224 w229] -> w173
        tunnel: w198 -> [w223 w229]
        tunnel: w190 -> [w222 _]
        tunnel: [w221 w228] -> w172
        tunnel: w197 -> [w220 w228]
        tunnel: [w219 w227] -> w171
        tunnel: w196 -> [w218 _]
        tunnel: w195 -> [w217 w227]
        frame False {
          n69 = Build Array (concatenate)(w223, w225) -> (w224:i32[])
          n70 = Build Array (concatenate)(w217, w218) -> (w219:i32[])
          n71 = Build Array (concatenate)(w220, w222) -> (w221:i32[])
          n72 = local write "Match?"(FALSE) -> ()
        }
        frame True {
          n73 = local write "Match?"(TRUE) -> ()
        }
      }
      n74 = case shown="참" "Save? (SP)" {
        tunnel: w169 -> [_ w207]
        tunnel: w163 -> [_ w206]
        tunnel: w159 -> [_ w204]
        frame False {
        }
        frame True {
          n75 = call "file_name_path_conv_sub.vi"("Add_No"=w206, "Add_Str"="Add_in Spectrum", "path_In"=w204) -> ("path_Out"=w208:path)  [unwired: 1 in]
          n76 = call-poly <vilib>:"Write Delimited Spreadsheet.vi"("file path (dialog if empty)"=w208, "format (%d)"="%d", "2D data"=w207, "delimiter (\\t)"="," ("delimiter (\\t)")) -> ()  [unwired: 10 in, 2 out]
        }
      }
      n77 = Build Array(w173, w172, w171) -> (w179:i32[][])
      n78 = Array Size(array=w179) -> (size(s)=w178:i32[])
      n79 = Index Array(array=w178, index=1) -> (element=w176:i32)
      "Errors(current)" <- w176
      n80 = Subtract(x=w170, y=w176) -> (x-y=w175:i32)
      n81 = Divide(x=w175, y=w170) -> (x/y=→"Accuracy(current)":dbl)
    }
    n82 = flat-sequence {
      tunnel: w82 -> [w130]
      tunnel: w81 -> [w129]
      tunnel: w80 -> [w128]
      tunnel: "Train No." -> [w123]
      tunnel: [w122] -> w85
      tunnel: w75 -> [w122]
      tunnel: [w121] -> w84
      tunnel: w74 -> [w121]
      tunnel: [w120] -> w70
      tunnel: w53 -> [w119]
      tunnel: [w118] -> w52
      tunnel: [w115] -> w43
      tunnel: w29 -> [w116]
      tunnel: w42 -> [w114]
      tunnel: w85 -> [w152]
      tunnel: w84 -> [w153]
      tunnel: w62 -> [w148]
      tunnel: "Train No." -> [w146]
      tunnel: w68 -> [w145]
      tunnel: w65 -> [w144]
      tunnel: w64 -> [w143]
      tunnel: [w138] -> w44
      tunnel: w43 -> [w138]
      frame #0 {
        n83 = Build Array(w130, w129, w128) -> (w115:i32[][])
        "Error list" <- w115
        n84 = Array Size(array=w115) -> (size(s)=w127:i32[])
        n85 = call "1Darray_sum_ave_optic_sub.vi"("1D array"=w119) -> ("Average"=w118:ext)  [unwired: 1 in, 1 out]
        n86 = case shown="참" "Save? (EL)" {
          tunnel: w115 -> [_ w134]
          tunnel: w116 -> [_ w132]
          tunnel: w114 -> [_ w131]
          frame False {
          }
          frame True {
            n87 = call "file_name_path_conv_sub.vi"("Add_No"=w131, "Add_Str"="Add_in Erorrs", "path_In"=w132) -> ("path_Out"=w135:path)  [unwired: 1 in]
            n88 = call-poly <vilib>:"Write Delimited Spreadsheet.vi"("file path (dialog if empty)"=w135, "format (%d)"="%d", "2D data"=w134, "delimiter (\\t)"="," ("delimiter (\\t)")) -> ()  [unwired: 10 in, 2 out]
          }
        }
        n89 = Index Array(array=w127, index=1) -> (element=w125:i32)
        "Errors" <- w125
        n90 = Subtract(x=w123, y=w125) -> (x-y=w124:i32)
        n91 = Divide(x=w124, y=w123) -> (x/y=w120:dbl)
        "Accuracy (prev)" <- w120
      }
      frame #1 {
        n92 = call "3D_to_2D_Sum_sub.vi"("3D array"=w152) -> ("2D_sum array"=w154:ext[][])
        n93 = call "2D_to_1D_Sum_sub.vi"("2D array"=w153) -> ("1D array"=w155:ext[])
        n94 = Divide(x=w154, y=w146) -> (x/y=w158:ext[][])
        n95 = Divide(x=w155, y=w146) -> (x/y=w157:ext[])
        n96 = Multiply(x=w158, y="Training rate") -> (x*y=w151:ext[][])
        n97 = Multiply(x=w157, y="Training rate") -> (x*y=w149:ext[])
        n98 = Transpose 2D Array(2D array=w151) -> (transposed array=w150:ext[][])
        n99 = call "file_name_path_conv_sub.vi"("Add_No"=w145, "Add_Str"=w144, "path_In"=w143) -> ("path_Out"=w140:path)  [unwired: 1 in]
        n100 = Build Array (concatenate)(w150, w149) -> (w147:ext[][])
        n101 = Subtract(x=w148, y=w147) -> (x-y=w139:ext[][])
        n102 = call-poly <vilib>:"Write Delimited Spreadsheet.vi"("file path (dialog if empty)"=w140, "format (%.3f)"="%d" ("format (%d)"), "2D data"=w139, "delimiter (\\t)"="," ("delimiter (\\t)")) -> ()  [unwired: 10 in, 2 out]
      }
    }
    n103 = Build Array (concatenate)(w51, w52) -> (w46:ext[])
    n104 = Add(x=w42, y=1) -> (x+y=w68:i32)
    n105 = Build Array (concatenate)(w71, w68) -> (w48:i32[])
    n106 = Build Array (concatenate)(w69, w70) -> (w47:dbl[])
    n107 = Bundle(w48, w46) -> (→"Loss":cluster{i32[], ext[]})  [unwired: 1 in]
    n108 = Bundle(w48, w47) -> (→"Accu":cluster{i32[], dbl[]})  [unwired: 1 in]
    n109 = Build Array(w48, w47, w46) -> (w41:ext[][])
    n110 = Transpose 2D Array(2D array=w41) -> (transposed array=w40:ext[][])
    n111 = case shown="참" "Save? (AL)" {
      tunnel: w40 -> [_ w103]
      tunnel: w29 -> [_ w100]
      frame False {
      }
      frame True {
        n112 = call "file_name_path_conv_sub.vi"("Add_No"=0, "Add_Str"="Add_in Acc&Loss", "path_In"=w100) -> ("path_Out"=w104:path)  [unwired: 1 in]
        n113 = call-poly <vilib>:"Write Delimited Spreadsheet.vi"("file path (dialog if empty)"=w104, "format (%.3f)"="%f" ("format (%d)"), "2D data"=w103, "delimiter (\\t)"="," ("delimiter (\\t)")) -> ()  [unwired: 10 in, 2 out]
      }
    }
    "epoch" <- w42
    "Loss" <- w52
  }
